vi "ReadCmdIn.vi"(0 "Connections":T1(array[cluster]), 2 "Log in":T2[](array[typedef]), 3 "Err in":path) -> (4 "data":string, 5 "Connections out":T1(array[cluster]), 6 "Log out":T2[](array[typedef]), 7 "Err out":path)   [LabVIEW 2012]
uses:
  <userlib>/ROSforLV/ROS/Code/Console/Servers/ServerSubs/ROSLog.ctl
  <userlib>/ROSforLV/ROS/Code/_ROSDefinition.vi
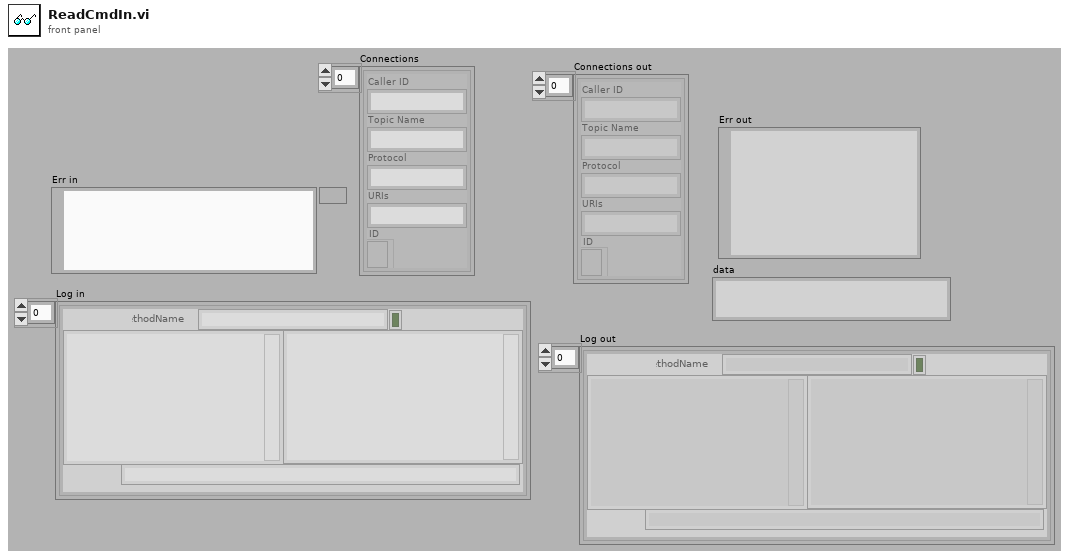
[diagram p1: front panel]
types:
  T1 = cluster{"Caller ID":string, "Topic Name":string, "Protocol":string, "URIs":string, "ID":refnum<k5>}[]
  T2 = typedef "ROSLog.ctl" = cluster{"Sent":string, "Reply":string, "MethodName":string, "success":bool, "Dir1":string, "Dir2":string, "Time Stamp":string, "error":errorcluster, "Preamble":string, "Midamble":string, "Postamble":string}
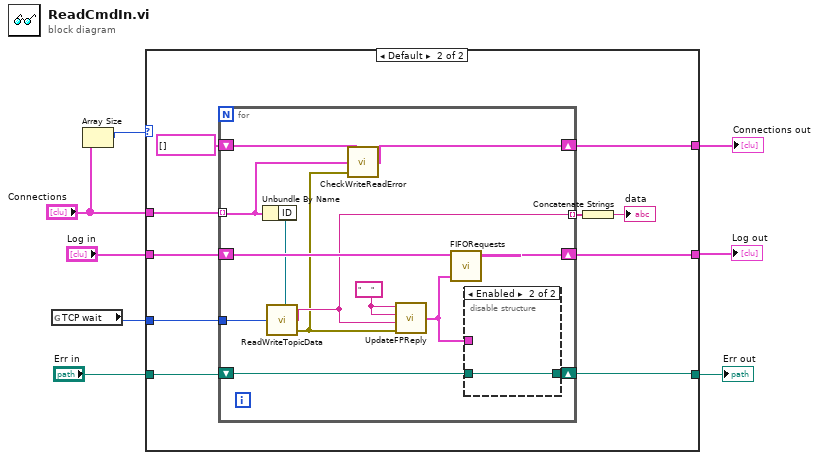
[diagram p0: block diagram]
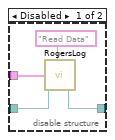
[diagram p3: hidden frame]
diagram:
  n1 = global read "_ROSDefinition.vi" "TCP wait"() -> (w1:i32)
  n2 = Array Size(array="Connections") -> (size(s)=w3:i32)
  n3 = case shown="Default" w3 {
    tunnel: [w11 w21] -> w8
    tunnel: "Log in" -> [w11 w20]
    tunnel: "Err in" -> [w10 w19]
    tunnel: [w10 w18] -> w5
    tunnel: "Connections" -> [w9 w17]
    tunnel: [w9 w14] -> w2
    tunnel: w1 -> [_ w12]
    frame 0 {
    }
    frame Default {
      n4 = for {
        shift-right: [w26] -> w18
        shift-left: w19 -> [w27]
        shift-right: [w33] -> w21
        shift-left: w20 -> [w34]
        tunnel: w17 -> [w31] mode=indexing
        tunnel: [w25] -> w16 mode=indexing
        shift-right: [w30] -> w14
        shift-left: T1 [] ("Connections out") -> [w29]
        tunnel: w12 -> [w28]
        w22 = "     " ("MethodName")
        n5 = Unbundle By Name(w31) -> ("ID"=w32:refnum<k5>)
        n6 = call <userlib>:"ReadWriteTopicData.vi"("timeout ms (1000)"=w28, "connection ID in"=w32) -> ("error out"=w24:errorcluster, "data out"=w25:string)  [unwired: 1 in, 1 out]
        n7 = call <userlib>:"CheckWriteReadError.vi"("error"=w24, "Subscriber in"=w31, "Connections in"=w29) -> ("Connections out"=w30:T1)
        n8 = call <userlib>:"UpdateFPReply.vi"("error in (no error)"=w24, "Reply"=w25, "Sent"=w22, "method"=w22) -> ("Log"=w23:T2)
        n9 = call <userlib>:"FIFORequests.vi"("Log"=w23, "Requests in"=w34) -> ("Requests out"=w33:T2[])  [unwired: 1 in]
        n10 = disable-structure shown="Enabled" {
          disable-tunnel: w27 -> [w38 w39]
          disable-tunnel: [w37 w39] -> w26
          disable-tunnel: w23 -> [w35 _]
          frame Disabled {
            n11 = call <userlib>:"RogersLog.vi"("Text to add"="Read Data", "Log"=w35, "LogPath in"=w38) -> ("LogPath out"=w37:path)  [unwired: 2 in, 1 out]
          }
          frame Enabled {
          }
        }
      }
      n12 = Concatenate Strings(w16) -> (→"data":string)
    }
  }
  "Log out" <- w8
  "Err out" <- w5
  "Connections out" <- w2
